vi "subvi_WcharToAscii.vi"(10 "Flattened whar IN":string) -> (2 "ASCII":string)   [LabVIEW 2020]
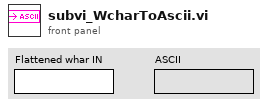
[diagram p1: front panel]
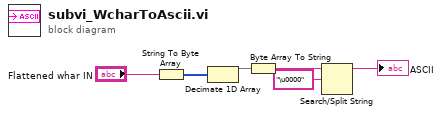
[diagram p0: block diagram]
diagram:
  n1 = String To Byte Array(string="Flattened whar IN") -> (unsigned byte array=w3:u8[])
  n2 = Decimate 1D Array(w3) -> (w4:u8[])  [unwired: 1 out]
  n3 = Byte Array To String(unsigned byte array=w4) -> (string=w5:string)
  n4 = Search/Split String(string=w5, search string/char (-)="\u0000") -> (substring before match=→"ASCII":string)  [unwired: 1 in, 2 out]
